vi "Get Aircraft Extra Data.vi"(8 "Error In":errorcluster, 11 "Aircraft ID":u8) -> (0 "Error Out":errorcluster, 3 "Extra Data Out":T1)   [LabVIEW 2014]
uses:
  Controls/Aircraft Extra Data.ctl
  MAVLink/Controls/MAVLink Optical Flow.ctl
  MAVLink/Controls/MAVLink EKF Status Report.ctl
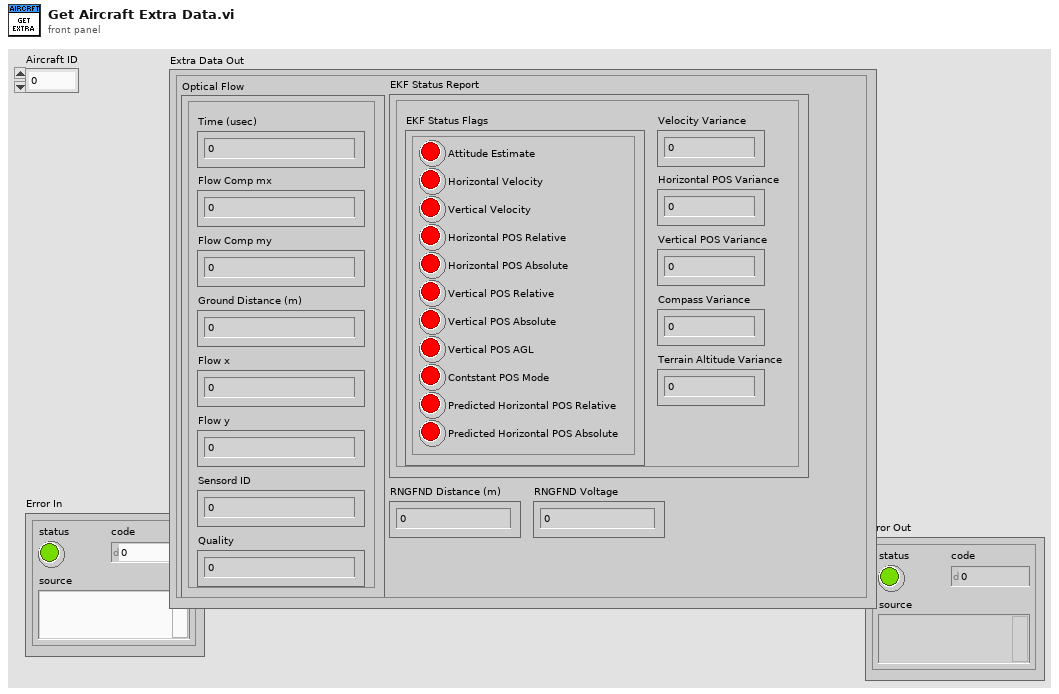
[diagram p1: front panel]
types:
  T1 = typedef "Aircraft Extra Data.ctl" = cluster{"Optical Flow":T2, "RNGFND Distance (m)":sgl, "RNGFND Voltage":sgl, "EKF Status Report":T3}
  T2 = typedef "MAVLink Optical Flow.ctl" = cluster{"Time (usec)":u64, "Flow Comp mx":sgl, "Flow Comp my":sgl, "Ground Distance (m)":sgl, "Flow x":i16, "Flow y":i16, "Sensord ID":u8, "Quality":u8}
  T3 = typedef "MAVLink EKF Status Report.ctl" = cluster{"EKF Status Flags":cluster{"Attitude Estimate":bool, "Horizontal Velocity":bool, "Vertical Velocity":bool, "Horizontal POS Relative":bool, "Horizontal POS Absolute":bool, "Vertical POS Relative":bool, "Vertical POS Absolute":bool, "Vertical POS AGL":bool, "Contstant POS Mode":bool, "Predicted Horizontal POS Relative":bool, "Predicted Horizontal POS Absolute":bool}, "Velocity Variance":sgl, "Horizontal POS Variance":sgl, "Vertical POS Variance":sgl, "Compass Variance":sgl, "Terrain Altitude Variance":sgl}
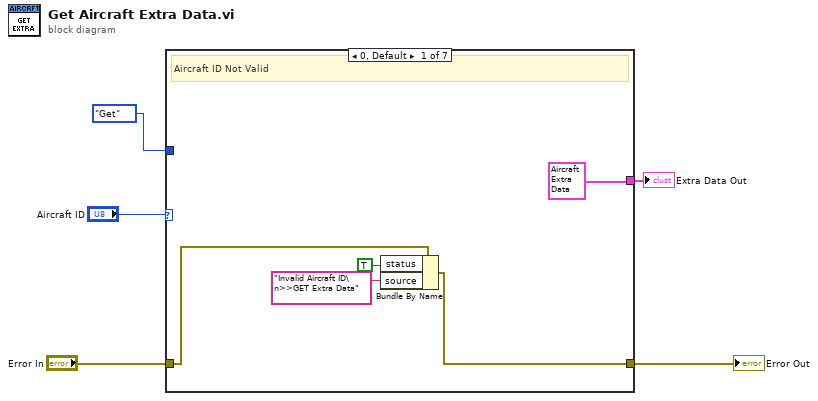
[diagram p0: block diagram]
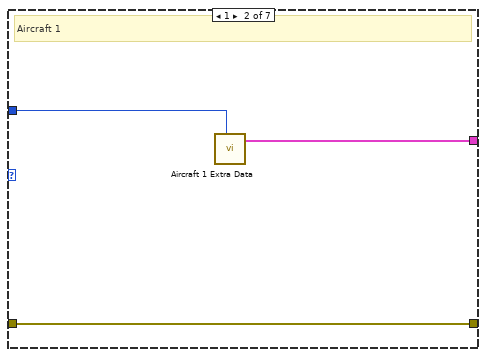
[diagram p2: hidden frame]
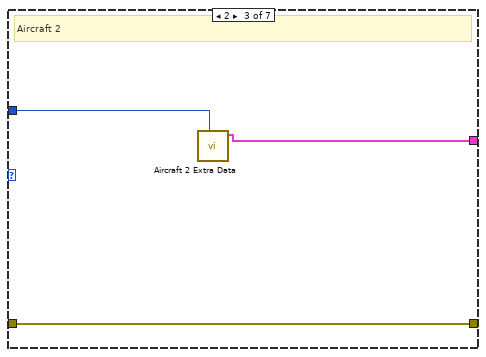
[diagram p3: hidden frame]
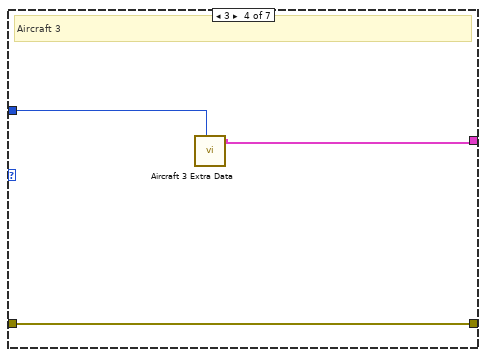
[diagram p4: hidden frame]
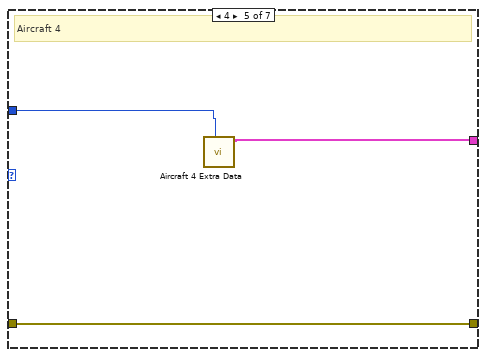
[diagram p5: hidden frame]
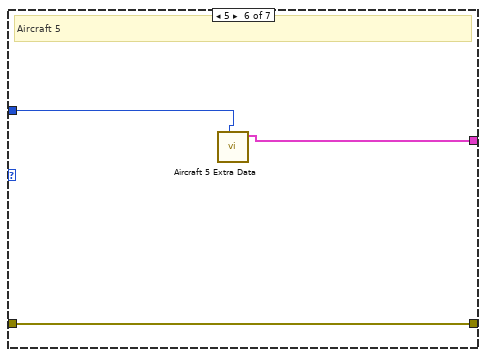
[diagram p6: hidden frame]
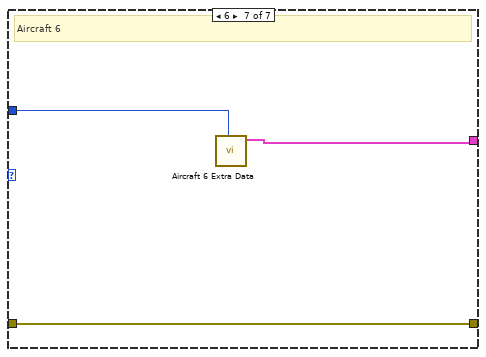
[diagram p7: hidden frame]
diagram:
  n1 = case shown="0, Default" "Aircraft ID" {
    tunnel: [T1 {"Optical Flow"={"Time (usec)"=0, "Flow Comp mx"=0.0, "Flow Comp my"=0.0, "Ground Distance (m)"=0.0, "Flow x"=0, "Flow y"=0, "Sensord ID"=0, "Quality"=0}, "RNGFND Distance (m)"=0.0, "RNGFND Voltage"=0.0, "EKF Status Report"={"EKF Status Flags"={"Attitude Estimate"=FALSE, "Horizontal Velocity"=FALSE, "Vertical Velocity"=FALSE, "Horizontal POS Relative"=FALSE, "Horizontal POS Absolute"=FALSE, "Vertical POS Relative"=FALSE, "Vertical POS Absolute"=FALSE, "Vertical POS AGL"=FALSE, "Contstant POS Mode"=FALSE, "Predicted Horizontal POS Relative"=FALSE, "Predicted Horizontal POS Absolute"=FALSE}, "Velocity Variance"=0.0, "Horizontal POS Variance"=0.0, "Vertical POS Variance"=0.0, "Compass Variance"=0.0, "Terrain Altitude Variance"=0.0}} ("Extra Data") w11 w15 w18 w21 w24 w27] -> w1
    tunnel: [w9 w13 w16 w19 w22 w25 w28] -> w4
    tunnel: "Error In" -> [w10 w13 w16 w19 w22 w25 w28]
    tunnel: enum16{"Get", "Set"}."Get" ("Method") -> [_ w12 w14 w17 w20 w23 w26]
    frame 0, Default {
      # "Aircraft ID Not Valid"
      n2 = Bundle By Name(cluster=w10, "status"=TRUE, "source"="Invalid Aircraft ID\n>>GET Extra Data") -> (w9:errorcluster)
    }
    frame 1 {
      # "Aircraft 1"
      n3 = call "Aircraft 1 Extra Data .vi"("Method"=w12) -> ("Extra Data Out"=w11:T1)  [unwired: 10 in]
    }
    frame 2 {
      # "Aircraft 2"
      n4 = call "Aircraft 2 Extra Data .vi"("Method"=w14) -> ("Extra Data Out"=w15:T1)  [unwired: 10 in]
    }
    frame 3 {
      # "Aircraft 3"
      n5 = call "Aircraft 3 Extra Data .vi"("Method"=w17) -> ("Extra Data Out"=w18:T1)  [unwired: 10 in]
    }
    frame 4 {
      # "Aircraft 4"
      n6 = call "Aircraft 4 Extra Data .vi"("Method"=w20) -> ("Extra Data Out"=w21:T1)  [unwired: 10 in]
    }
    frame 5 {
      # "Aircraft 5"
      n7 = call "Aircraft 5 Extra Data .vi"("Method"=w23) -> ("Extra Data Out"=w24:T1)  [unwired: 10 in]
    }
    frame 6 {
      # "Aircraft 6"
      n8 = call "Aircraft 6 Extra Data .vi"("Method"=w26) -> ("Extra Data Out"=w27:T1)  [unwired: 10 in]
    }
  }
  "Error Out" <- w4
  "Extra Data Out" <- w1
